vi "GetMultitoneFrequency.vi"(7 "Selection":u8(ring) items=["Value", "Minimum", "Maximum"], 8 "error in (no error)":errorcluster, 9 "Tone Index":u16(ring) items=["Tone 1", "Tone 2", "Tone 3", "Tone 4", "Tone 5", "Tone 6", "Tone 7", "Tone 8", "Tone 9", "Tone 10"], 10 "ParamWave Name":string, 11 "VISA resource name":refnum<visa-resource-name>) -> (0 "error out":errorcluster, 2 "Frequency [Hz]":dbl, 3 "VISA resource name out":refnum<visa-resource-name>)   [LabVIEW 2020, in "Active Technologies AWG3000.lvlib"]
uses:
  Active Technologies AWG3000.lvlib
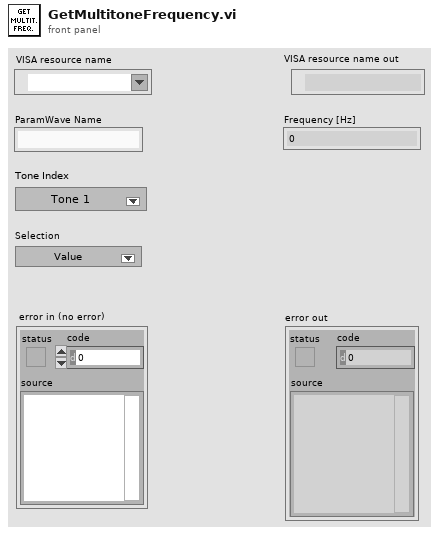
[diagram p1: front panel]
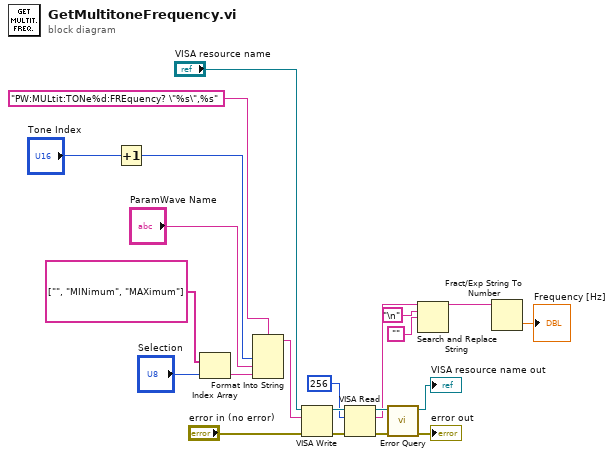
[diagram p0: block diagram]
diagram:
  n1 = Increment(x="Tone Index") -> (x+1=w1:u16)
  n2 = Index Array(array=string[] ["", "MINimum", "MAXimum"], index="Selection") -> (element=w4:string)
  n3 = Format Into String(format string="PW:MULtit:TONe%d:FREquency? \"%s\",%s" ("write buffer"), w1, "ParamWave Name", w4) -> (resulting string=w5:string)  [unwired: 2 in, 1 out]
  n4 = VISA Write(VISA resource name="VISA resource name", write buffer=w5, error in (no error)="error in (no error)") -> (VISA resource name out=w19:refnum<visa-resource-name>, error out=w18:errorcluster)  [unwired: 1 out]
  n5 = VISA Read(VISA resource name=w19, byte count=u32 256, error in (no error)=w18) -> (VISA resource name out=w16:refnum<visa-resource-name>, read buffer=w6:string, error out=w15:errorcluster)  [unwired: 1 out]
  n6 = call "Error Query.vi"("error in (no error)"=w15, "VISA resource name"=w16) -> ("error out"=→"error out":errorcluster, "VISA resource name out"=→"VISA resource name out":refnum<visa-resource-name>)  [unwired: 6 in, 2 out]
  n7 = Search and Replace String(input string=w6, search string="\n", replace string="") -> (result string=w9:string)  [unwired: 5 in, 3 out]
  n8 = Fract/Exp String To Number(string=w9) -> (number=→"Frequency [Hz]":dbl)  [unwired: 3 in, 1 out]
